vi "Global Encoder.vi"() -> ()   [LabVIEW 2017]
panel:
  out "Count Encoder 2":dbl
  out "Count Encoder 1":dbl
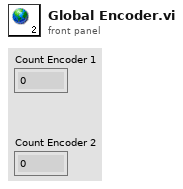
[diagram p1: front panel]
diagram:
